vi "Write Payload.vi"(10 "Payload":string, 11 "GDSII.DataType.Bit Array in":refnum<class "GDSII.DataType.Bit Array.lvclass">) -> (3 "GDSII.DataType.Bit Array out":refnum<class "GDSII.DataType.Bit Array.lvclass">)   [LabVIEW 2019, in "GDSII.DataType.Bit Array.lvclass"]
uses:
  GDSII.DataType.Bit Array.lvclass
  GDSII.DataType.Bit Array.lvclass/GDSII.DataType.Bit Array.ctl
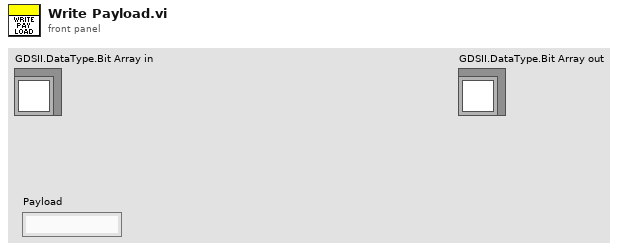
[diagram p1: front panel]
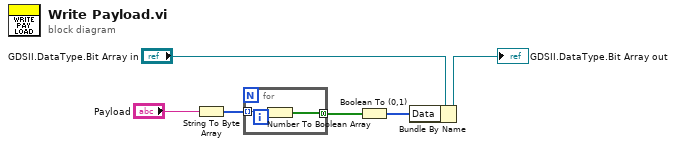
[diagram p0: block diagram]
diagram:
  n1 = String To Byte Array(string="Payload") -> (unsigned byte array=w6:u8[])
  n2 = for {
    tunnel: w6 -> [w8] mode=indexing
    tunnel: [w7] -> w5 mode=concatenating
    n3 = Number To Boolean Array(number=w8) -> (Boolean array=w7:bool[])
  }
  n4 = Boolean To (0,1)(Boolean=w5) -> (0, 1=w1:i16[])
  n5 = Bundle By Name(cluster="GDSII.DataType.Bit Array in", "Data"=w1) -> (→"GDSII.DataType.Bit Array out":refnum<class "GDSII.DataType.Bit Array.lvclass">)
